vi "HIOKI PW3390 Configuration Phase Correct.vi"() -> ()   [LabVIEW 2009]
doc: "Sets the phase correction for current sensors."
uses:
  <instrlib>/PW3390/Common/_Initialize/HIOKI PW3390 Initialize LAN.vi
  <instrlib>/PW3390/Common/_Initialize/HIOKI PW3390 Initialize RS-232C.vi
panel:
  out "error out":errorcluster
  in  "Communication Interface":enum16{"LAN", "RS-232C"}(ring)
  in  "COM Port":refnum<visa-resource-name>="COM1"
  in  "baud rate (38400bps)":u32=38400
  in  "IP Address":string="192.168.1.1"
  in  "Phase Correct":T1(array[ring])=[enum."OFF", enum."OFF", enum."OFF", enum."OFF"]
  # "CH1"
  # "CH2"
  # "CH3"
  # "CH4"
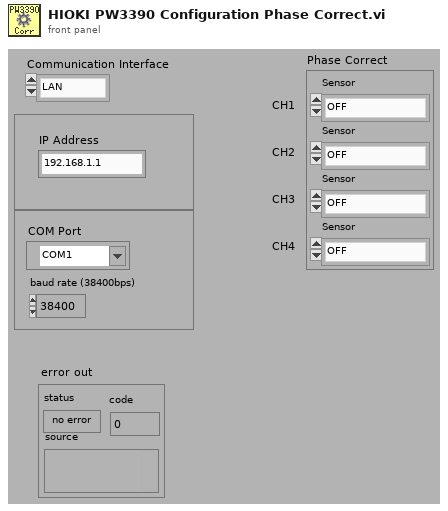
[diagram p1: front panel]
types:
  T1 = enum16{"OFF", "CT6841", "CT6843", "CT6844", "CT6845", "CT6846", "CT6862", "CT6863", "CT6865", "9709", "PW9100", "9272-05 (20A)", "9272-05 (200A)", "CT7044", "CT7045", "CT7046", "CT7642", "CT7742"}[]
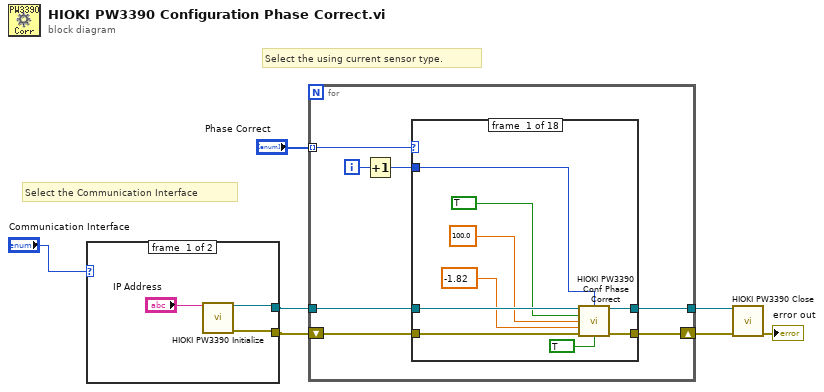
[diagram p0: block diagram]
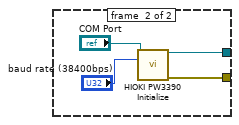
[diagram p2: hidden frame]
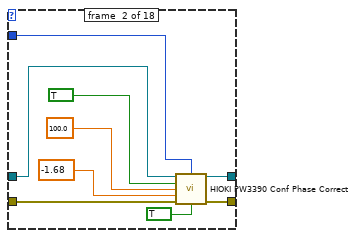
[diagram p3: hidden frame]
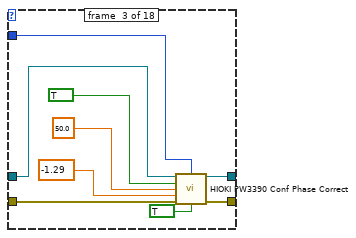
[diagram p4: hidden frame]
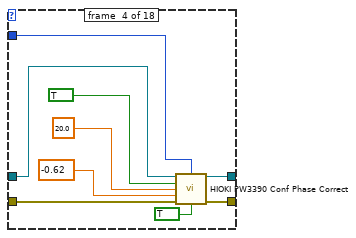
[diagram p5: hidden frame]
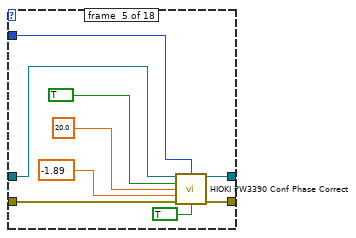
[diagram p6: hidden frame]
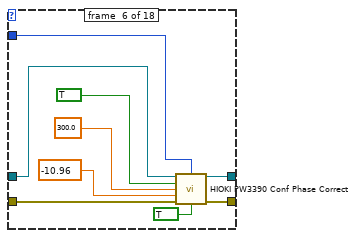
[diagram p7: hidden frame]
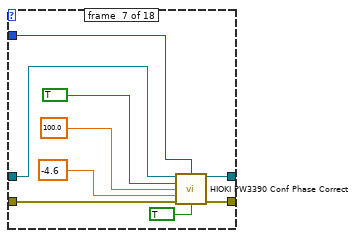
[diagram p8: hidden frame]
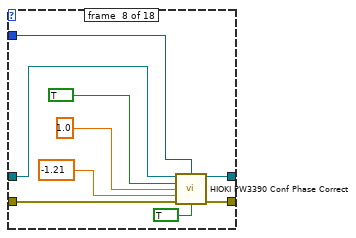
[diagram p9: hidden frame]
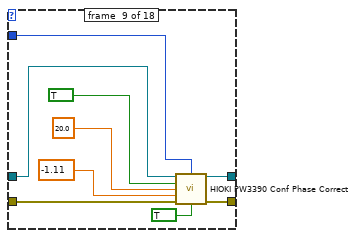
[diagram p10: hidden frame]
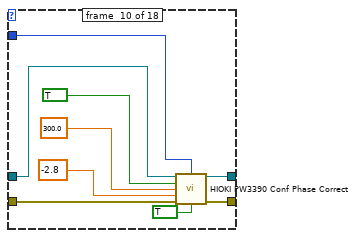
[diagram p11: hidden frame]
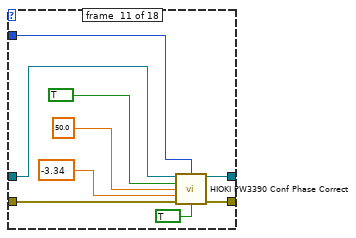
[diagram p12: hidden frame]
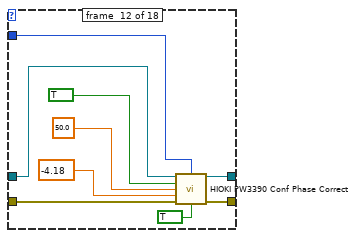
[diagram p13: hidden frame]
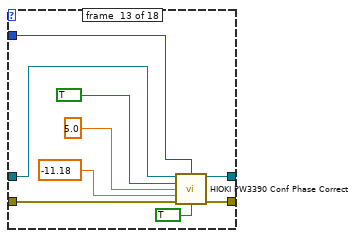
[diagram p14: hidden frame]
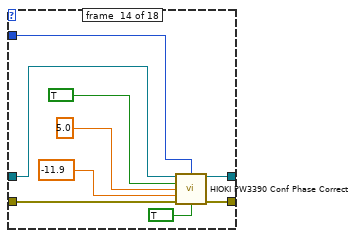
[diagram p15: hidden frame]
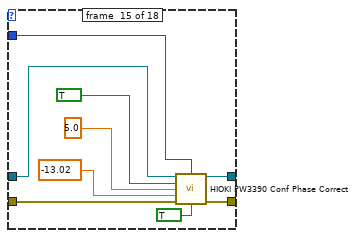
[diagram p16: hidden frame]
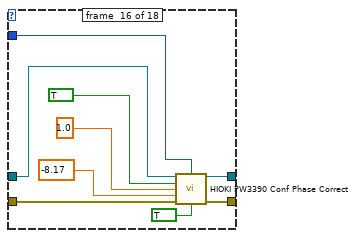
[diagram p17: hidden frame]
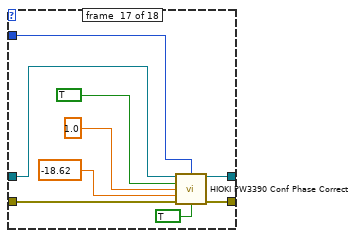
[diagram p18: hidden frame]
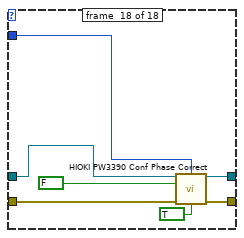
[diagram p19: hidden frame]
diagram:
  # "Select the Communication Interface"
  # "Select the using current sensor type."
  n1 = case shown="\"LAN\", デフォルト" "Communication Interface" {
    tunnel: [w9 w14] -> w5
    tunnel: [w8 w13] -> w4
    frame #0 {
      n2 = call-poly <instrlib>:"HIOKI PW3390 Initialize.vi"("IP Address"="IP Address") -> ("VISA Resource out"=w9:refnum<visa-resource-name>, "error out"=w8:errorcluster)  [unwired: 12 in, 1 out]
    }
    frame #1 {
      n3 = call-poly <instrlib>:"HIOKI PW3390 Initialize.vi"("COM Port"="COM Port", "baud rate (38400bps)"="baud rate (38400bps)") -> ("VISA Resource out"=w14:refnum<visa-resource-name>, "error out"=w13:errorcluster)  [unwired: 11 in, 1 out]
    }
  }
  n4 = for {
    tunnel: "Phase Correct" -> [w17] mode=indexing
    tunnel: w5 -> [w16]
    tunnel: [w19] -> w3
    shift-right: [w18] -> w2
    shift-left: w4 -> [w15]
    i -> [w21]
    n5 = Increment(x=w21) -> (x+1=w20:i32)
    n6 = case shown="\"CT6841\", デフォルト" w17 {
      tunnel: w20 -> [w29 w39 w48 w57 w66 w75 w82 w93 w102 w111 w120 w129 w138 w147 w156 w165 w174 w181]
      tunnel: [w28 w38 w46 w56 w65 w72 w81 w92 w101 w110 w119 w128 w137 w146 w155 w164 w173 w180] -> w19
      tunnel: [w27 w37 w45 w55 w64 w71 w80 w91 w100 w109 w118 w127 w136 w145 w154 w163 w172 w179] -> w18
      tunnel: w16 -> [w30 w36 w47 w54 w62 w74 w84 w89 w98 w107 w116 w125 w135 w144 w152 w161 w170 w177]
      tunnel: w15 -> [w26 w35 w44 w53 w63 w73 w83 w90 w99 w108 w117 w126 w134 w143 w153 w162 w171 w178]
      frame #0 {
        n7 = call <instrlib>:"HIOKI PW3390 Conf Phase Correct.vi"("VISA Resource"=w30, "CH (1)"=w29, "Correct (F: OFF)"=TRUE, "Frequency (kHz) (100.000)"=100.0, "Angle (0.00)"=-1.82, "error in (no error)"=w26, "Error Out (F: Off)"=TRUE) -> ("VISA Resource out"=w28:refnum<visa-resource-name>, "error out"=w27:errorcluster)  [unwired: 4 in, 3 out]
      }
      frame #1 {
        n8 = call <instrlib>:"HIOKI PW3390 Conf Phase Correct.vi"("VISA Resource"=w36, "CH (1)"=w39, "Correct (F: OFF)"=TRUE, "Frequency (kHz) (100.000)"=100.0, "Angle (0.00)"=-1.68, "error in (no error)"=w35, "Error Out (F: Off)"=TRUE) -> ("VISA Resource out"=w38:refnum<visa-resource-name>, "error out"=w37:errorcluster)  [unwired: 4 in, 3 out]
      }
      frame #2 {
        n9 = call <instrlib>:"HIOKI PW3390 Conf Phase Correct.vi"("VISA Resource"=w47, "CH (1)"=w48, "Correct (F: OFF)"=TRUE, "Frequency (kHz) (100.000)"=50.0, "Angle (0.00)"=-1.29, "error in (no error)"=w44, "Error Out (F: Off)"=TRUE) -> ("VISA Resource out"=w46:refnum<visa-resource-name>, "error out"=w45:errorcluster)  [unwired: 4 in, 3 out]
      }
      frame #3 {
        n10 = call <instrlib>:"HIOKI PW3390 Conf Phase Correct.vi"("VISA Resource"=w54, "CH (1)"=w57, "Correct (F: OFF)"=TRUE, "Frequency (kHz) (100.000)"=20.0, "Angle (0.00)"=-0.62, "error in (no error)"=w53, "Error Out (F: Off)"=TRUE) -> ("VISA Resource out"=w56:refnum<visa-resource-name>, "error out"=w55:errorcluster)  [unwired: 4 in, 3 out]
      }
      frame #4 {
        n11 = call <instrlib>:"HIOKI PW3390 Conf Phase Correct.vi"("VISA Resource"=w62, "CH (1)"=w66, "Correct (F: OFF)"=TRUE, "Frequency (kHz) (100.000)"=20.0, "Angle (0.00)"=-1.89, "error in (no error)"=w63, "Error Out (F: Off)"=TRUE) -> ("VISA Resource out"=w65:refnum<visa-resource-name>, "error out"=w64:errorcluster)  [unwired: 4 in, 3 out]
      }
      frame #5 {
        n12 = call <instrlib>:"HIOKI PW3390 Conf Phase Correct.vi"("VISA Resource"=w74, "CH (1)"=w75, "Correct (F: OFF)"=TRUE, "Frequency (kHz) (100.000)"=300.0, "Angle (0.00)"=-10.96, "error in (no error)"=w73, "Error Out (F: Off)"=TRUE) -> ("VISA Resource out"=w72:refnum<visa-resource-name>, "error out"=w71:errorcluster)  [unwired: 4 in, 3 out]
      }
      frame #6 {
        n13 = call <instrlib>:"HIOKI PW3390 Conf Phase Correct.vi"("VISA Resource"=w84, "CH (1)"=w82, "Correct (F: OFF)"=TRUE, "Frequency (kHz) (100.000)"=100.0, "Angle (0.00)"=-4.6, "error in (no error)"=w83, "Error Out (F: Off)"=TRUE) -> ("VISA Resource out"=w81:refnum<visa-resource-name>, "error out"=w80:errorcluster)  [unwired: 4 in, 3 out]
      }
      frame #7 {
        n14 = call <instrlib>:"HIOKI PW3390 Conf Phase Correct.vi"("VISA Resource"=w89, "CH (1)"=w93, "Correct (F: OFF)"=TRUE, "Frequency (kHz) (100.000)"=1.0, "Angle (0.00)"=-1.21, "error in (no error)"=w90, "Error Out (F: Off)"=TRUE) -> ("VISA Resource out"=w92:refnum<visa-resource-name>, "error out"=w91:errorcluster)  [unwired: 4 in, 3 out]
      }
      frame #8 {
        n15 = call <instrlib>:"HIOKI PW3390 Conf Phase Correct.vi"("VISA Resource"=w98, "CH (1)"=w102, "Correct (F: OFF)"=TRUE, "Frequency (kHz) (100.000)"=20.0, "Angle (0.00)"=-1.11, "error in (no error)"=w99, "Error Out (F: Off)"=TRUE) -> ("VISA Resource out"=w101:refnum<visa-resource-name>, "error out"=w100:errorcluster)  [unwired: 4 in, 3 out]
      }
      frame #9 {
        n16 = call <instrlib>:"HIOKI PW3390 Conf Phase Correct.vi"("VISA Resource"=w107, "CH (1)"=w111, "Correct (F: OFF)"=TRUE, "Frequency (kHz) (100.000)"=300.0, "Angle (0.00)"=-2.8, "error in (no error)"=w108, "Error Out (F: Off)"=TRUE) -> ("VISA Resource out"=w110:refnum<visa-resource-name>, "error out"=w109:errorcluster)  [unwired: 4 in, 3 out]
      }
      frame #10 {
        n17 = call <instrlib>:"HIOKI PW3390 Conf Phase Correct.vi"("VISA Resource"=w116, "CH (1)"=w120, "Correct (F: OFF)"=TRUE, "Frequency (kHz) (100.000)"=50.0, "Angle (0.00)"=-3.34, "error in (no error)"=w117, "Error Out (F: Off)"=TRUE) -> ("VISA Resource out"=w119:refnum<visa-resource-name>, "error out"=w118:errorcluster)  [unwired: 4 in, 3 out]
      }
      frame #11 {
        n18 = call <instrlib>:"HIOKI PW3390 Conf Phase Correct.vi"("VISA Resource"=w125, "CH (1)"=w129, "Correct (F: OFF)"=TRUE, "Frequency (kHz) (100.000)"=50.0, "Angle (0.00)"=-4.18, "error in (no error)"=w126, "Error Out (F: Off)"=TRUE) -> ("VISA Resource out"=w128:refnum<visa-resource-name>, "error out"=w127:errorcluster)  [unwired: 4 in, 3 out]
      }
      frame #12 {
        n19 = call <instrlib>:"HIOKI PW3390 Conf Phase Correct.vi"("VISA Resource"=w135, "CH (1)"=w138, "Correct (F: OFF)"=TRUE, "Frequency (kHz) (100.000)"=5.0, "Angle (0.00)"=-11.18, "error in (no error)"=w134, "Error Out (F: Off)"=TRUE) -> ("VISA Resource out"=w137:refnum<visa-resource-name>, "error out"=w136:errorcluster)  [unwired: 4 in, 3 out]
      }
      frame #13 {
        n20 = call <instrlib>:"HIOKI PW3390 Conf Phase Correct.vi"("VISA Resource"=w144, "CH (1)"=w147, "Correct (F: OFF)"=TRUE, "Frequency (kHz) (100.000)"=5.0, "Angle (0.00)"=-11.9, "error in (no error)"=w143, "Error Out (F: Off)"=TRUE) -> ("VISA Resource out"=w146:refnum<visa-resource-name>, "error out"=w145:errorcluster)  [unwired: 4 in, 3 out]
      }
      frame #14 {
        n21 = call <instrlib>:"HIOKI PW3390 Conf Phase Correct.vi"("VISA Resource"=w152, "CH (1)"=w156, "Correct (F: OFF)"=TRUE, "Frequency (kHz) (100.000)"=5.0, "Angle (0.00)"=-13.02, "error in (no error)"=w153, "Error Out (F: Off)"=TRUE) -> ("VISA Resource out"=w155:refnum<visa-resource-name>, "error out"=w154:errorcluster)  [unwired: 4 in, 3 out]
      }
      frame #15 {
        n22 = call <instrlib>:"HIOKI PW3390 Conf Phase Correct.vi"("VISA Resource"=w161, "CH (1)"=w165, "Correct (F: OFF)"=TRUE, "Frequency (kHz) (100.000)"=1.0, "Angle (0.00)"=-8.17, "error in (no error)"=w162, "Error Out (F: Off)"=TRUE) -> ("VISA Resource out"=w164:refnum<visa-resource-name>, "error out"=w163:errorcluster)  [unwired: 4 in, 3 out]
      }
      frame #16 {
        n23 = call <instrlib>:"HIOKI PW3390 Conf Phase Correct.vi"("VISA Resource"=w170, "CH (1)"=w174, "Correct (F: OFF)"=TRUE, "Frequency (kHz) (100.000)"=1.0, "Angle (0.00)"=-18.62, "error in (no error)"=w171, "Error Out (F: Off)"=TRUE) -> ("VISA Resource out"=w173:refnum<visa-resource-name>, "error out"=w172:errorcluster)  [unwired: 4 in, 3 out]
      }
      frame #17 {
        n24 = call <instrlib>:"HIOKI PW3390 Conf Phase Correct.vi"("VISA Resource"=w177, "CH (1)"=w181, "Correct (F: OFF)"=FALSE, "error in (no error)"=w178, "Error Out (F: Off)"=TRUE) -> ("VISA Resource out"=w180:refnum<visa-resource-name>, "error out"=w179:errorcluster)  [unwired: 6 in, 3 out]
      }
    }
  }
  n25 = call <instrlib>:"HIOKI PW3390 Close.vi"("VISA Resource"=w3, "error in (no error)"=w2) -> ("error out"=→"error out":errorcluster)  [unwired: 13 in]
